vi "Dashboard globals.vi"() -> ()   [LabVIEW 2018]
panel:
  in  "Right y coordinate":sgl
  in  "Right x coordinate":sgl
  in  "Left y coordinate":sgl
  in  "Left x coordinate":sgl
  in  "Center y coordinate":sgl
  in  "Center x coordinate":sgl
  out "Desired Target":T1(radio)=enum."Rocket or Loading Station"
  in  "Enable Vision\nProcessing":bool
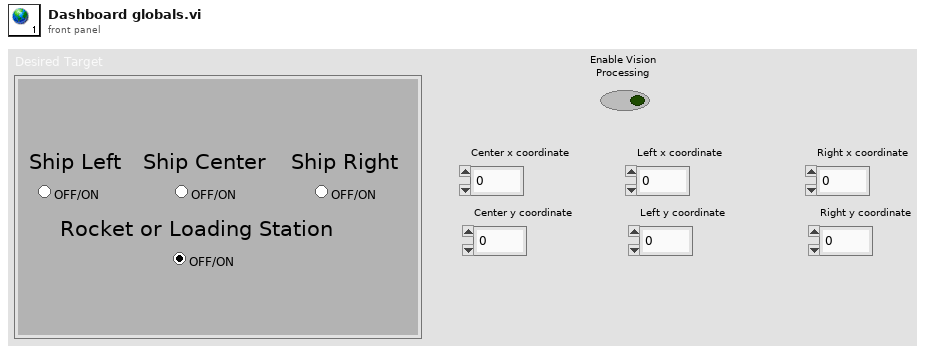
[diagram p1: front panel]
types:
  T1 = enum32{"Ship Left", "Ship Center", "Ship Right", "Rocket or Loading Station"}
diagram:
